vi "get_averaging_params_fd.vi"(10 "Modulation info":T3 {"Hi channels at low" min=0 step=1; "Low carriers" format="%#_6p"; "High carriers" format="%#_6p"}, 11 "Config":T4={"I/O"={"Format"={"Rate"=4, "Bits"=32, "Channels"=2}, "card #"=1, "# buffers"=96000}, "High rate STFT"={"Win param"=101.5, "Window type"=61, "Win order"=2, "DFT size"=64, "Channels"=[7], "Oversample"=64}, "Low rate STFT"={"Win param"=120.0, "Window type"=61, "Win order"=8, "DFT size"=64, "Channels"=[7], "Oversample"=64}, "Filtering"={"Hum"={"Frequency"=0.0, "Tc"=0.0, "Limit"=101.5, "FFT filter"=FALSE, "Detrend mode"=enum."Robust linear", "Enable"=FALSE}, "Kalman"={"Process noise"=101.5, "Measure noise"=101.5, "Unlock m noise"=101.5, "Mode"=enum."FFT"}, "Distortion"={"LF cut"=101.5, "Tc"=3.0, "Limit"=101.5, "FFT filter"=FALSE, "Detrend mode"=enum."Robust linear", "Enable"=FALSE}, "Lowpass"={"Frequency"=0.0, "Order"=0, "Enable"=FALSE}, "Impulse"={"Win order"=102, "Locked limit"=101.5, "Locked count"=102, "Threshold Tc"=101.5, "Thresh sigmas"=101.5, "Thresh min"=101.5, "After"=0, "Detrend"=FALSE, "Enable"=FALSE}}} {"Filtering"."Impulse"."Thresh min" format="%#_3p"; "Filtering"."Impulse"."Threshold Tc" format="%#_3p"; "Filtering"."Impulse"."Locked limit" format="%#_3p"; "Filtering"."Impulse"."Thresh sigmas" format="%#_3p"; "Filtering"."Lowpass"."Frequency" format="%#_4p"; "Filtering"."Distortion"."Limit" format="%#_3p"; "Filtering"."Distortion"."LF cut" format="%#_3p"; "Filtering"."Kalman"."Unlock m noise" format="%#_3p"; "Filtering"."Kalman"."Measure noise" format="%#_3p"; "Filtering"."Kalman"."Process noise" format="%#_3p"; "Filtering"."Hum"."Limit" format="%#_3p"; "Filtering"."Hum"."Frequency" format="%#_4p"; "Low rate STFT"."Oversample" min=1 step=1; "Low rate STFT"."Channels" min=0 step=1; "Low rate STFT"."DFT size" min=1 step=1; "Low rate STFT"."Window type" items=["Rectangle"=0, "Hanning"=1, "Hamming"=2, "Blackman-Harris"=3, "Exact Blackman"=4, "Blackman"=5, "Flat Top"=6, "4 Term B-Harris "=7, "7 Term B-Harris"=8, "Low Sidelobe"=9, "Blackman Nuttall"=11, "Triangle"=30, "Bartlett-Hanning"=31, "Bohman"=32, "Parzen"=33, "Welch"=34, "Kaiser"=60, "Dolph-Chebyshev"=61, "Gaussian"=62]; "High rate STFT"."Oversample" min=1 step=1; "High rate STFT"."Channels" min=0 step=1; "High rate STFT"."DFT size" min=1 step=1; "High rate STFT"."Window type" items=["Rectangle"=0, "Hanning"=1, "Hamming"=2, "Blackman-Harris"=3, "Exact Blackman"=4, "Blackman"=5, "Flat Top"=6, "4 Term B-Harris "=7, "7 Term B-Harris"=8, "Low Sidelobe"=9, "Blackman Nuttall"=11, "Triangle"=30, "Bartlett-Hanning"=31, "Bohman"=32, "Parzen"=33, "Welch"=34, "Kaiser"=60, "Dolph-Chebyshev"=61, "Gaussian"=62]}) -> (2 "Hum params":T1={"Order"=0, "Time constant"=0.0, "Detrend mode"=enum."Robust linear", "TD amplitude limit"=inf, "FFT filter"=TRUE, "Notch channels"=[], "LF cutoff"=0, "FD amplitude limit"=0.0}, 3 "Distortion params":T1={"Order"=0, "Time constant"=0.0, "Detrend mode"=enum."Robust linear", "TD amplitude limit"=inf, "FFT filter"=TRUE, "Notch channels"=[], "LF cutoff"=0, "FD amplitude limit"=0.0})   [LabVIEW 2014]
uses:
  averaging_filter_params.ctl
  detrend_mode.ctl
  ilemt_config.ctl
  io_config.ctl
  stft_params.ctl
  <vilib>/Analysis/4window.llb/windowTd.ctl
  filter_params.ctl
  modulation_info.ctl
  <vilib>/Analysis/NI_AALPro.lvlib
panel:
  # "Get averaging filter parameters for the distortion and hum filters,\noperating at Fd demodulated output rate."
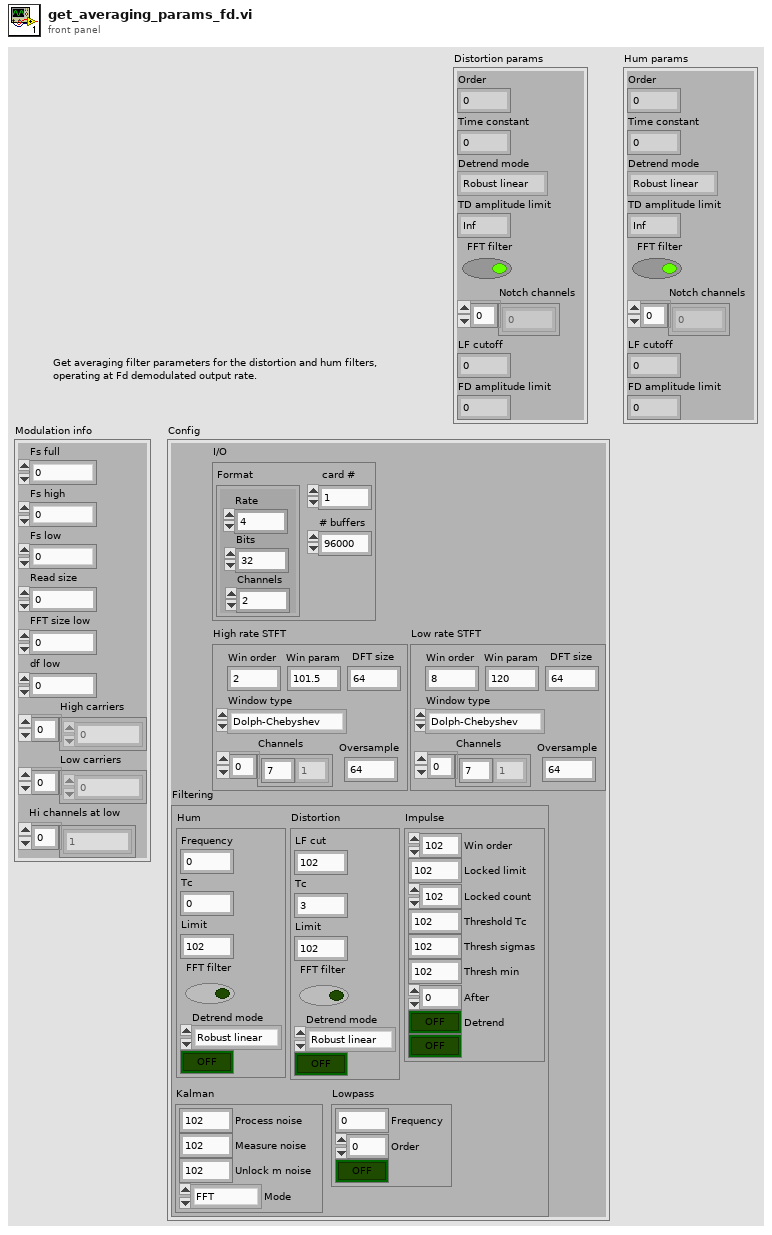
[diagram p1: front panel]
types:
  T1 = typedef "averaging_filter_params.ctl" = cluster{"Order":i32, "Time constant":dbl, "Detrend mode":T2, "TD amplitude limit":dbl, "FFT filter":bool, "Notch channels":i32[], "LF cutoff":i32, "FD amplitude limit":dbl}
  T2 = typedef "detrend_mode.ctl" = enum16{"Zero mean", "Linear", "Robust linear"}
  T3 = typedef "modulation_info.ctl" = cluster{"Fs full":dbl, "Fs high":dbl, "Fs low":dbl, "Read size":i32, "FFT size low":i32, "df low":dbl, "High carriers":dbl[], "Low carriers":dbl[], "Hi channels at low":i32[]}
  T4 = typedef "ilemt_config.ctl" = cluster{"I/O":T5, "High rate STFT":T6, "Low rate STFT":T6, "Filtering":T8}
  T5 = typedef "io_config.ctl" = cluster{"Format":cluster{"Rate":i32, "Bits":i32, "Channels":u32}, "card #":u32, "# buffers":i32}
  T6 = typedef "stft_params.ctl" = cluster{"Win param":dbl, "Window type":T7, "Win order":i32, "DFT size":i32, "Channels":i32[], "Oversample":i32}
  T7 = typedef "NI_AALPro.lvlib/windowTd.ctl" = u32
  T8 = typedef "filter_params.ctl" = cluster{"Hum":cluster{"Frequency":dbl, "Tc":dbl, "Limit":dbl, "FFT filter":bool, "Detrend mode":T2, "Enable":bool}, "Kalman":cluster{"Process noise":dbl, "Measure noise":dbl, "Unlock m noise":dbl, "Mode":enum16{"FFT", "KF demod"}}, "Distortion":cluster{"LF cut":dbl, "Tc":dbl, "Limit":dbl, "FFT filter":bool, "Detrend mode":T2, "Enable":bool}, "Lowpass":cluster{"Frequency":dbl, "Order":i32, "Enable":bool}, "Impulse":cluster{"Win order":i32, "Locked limit":dbl, "Locked count":i32, "Threshold Tc":dbl, "Thresh sigmas":dbl, "Thresh min":dbl, "After":i32, "Detrend":bool, "Enable":bool}}
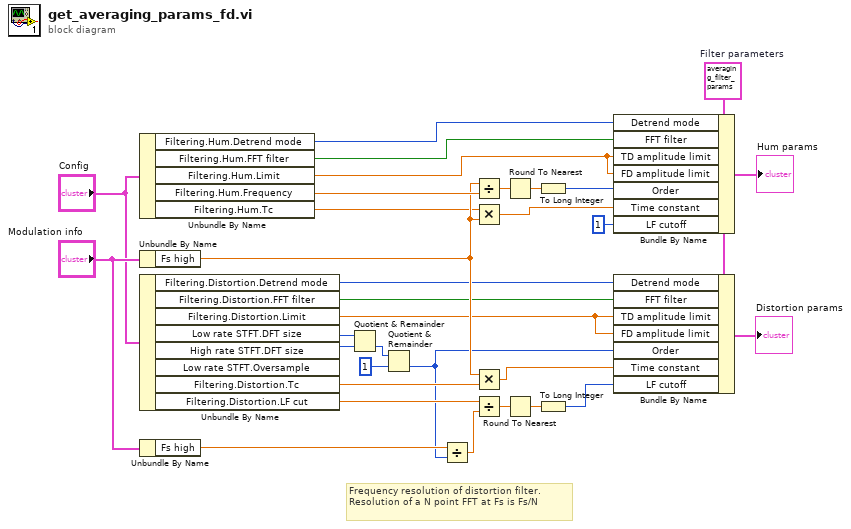
[diagram p0: block diagram]
diagram:
  w15 = T1 {"Order"=0, "Time constant"=0.0, "Detrend mode"=enum."Robust linear", "TD amplitude limit"=inf, "FFT filter"=TRUE, "Notch channels"=[], "LF cutoff"=0, "FD amplitude limit"=inf}  # Filter parameters
  # "Frequency resolution of distortion filter.   Resolution of a N point FFT at Fs is Fs/N"
  n1 = Unbundle By Name("Config") -> ("Filtering.Hum.Detrend mode"=w7:T2, "Filtering.Hum.FFT filter"=w8:bool, "Filtering.Hum.Limit"=w9:dbl, "Filtering.Hum.Frequency"=w30:dbl, "Filtering.Hum.Tc"=w18:dbl)
  n2 = Unbundle By Name("Modulation info") -> ("Fs high"=w26:dbl)
  n3 = Unbundle By Name("Config") -> ("Filtering.Distortion.Detrend mode"=w5:T2, "Filtering.Distortion.FFT filter"=w4:bool, "Filtering.Distortion.Limit"=w6:dbl, "Low rate STFT.DFT size"=w14:i32, "High rate STFT.DFT size"=w13:i32, "Filtering.Distortion.Tc"=w27:dbl, "Filtering.Distortion.LF cut"=w22:dbl)  [unwired: 1 out]
  n4 = Unbundle By Name("Modulation info") -> ("Fs high"=w11:dbl)
  n5 = Quotient & Remainder(x=w14, y=w13) -> (floor(x/y)=w3:i32)  [unwired: 1 out]
  n6 = Quotient & Remainder(x=w3, y=1) -> (floor(x/y)=w2:i32)  [unwired: 1 out]
  n7 = Divide(x=w11, y=w2) -> (x/y=w10:dbl)
  n8 = Divide(x=w26, y=w30) -> (x/y=w17:dbl)
  n9 = Multiply(x=w18, y=w26) -> (x*y=w25:dbl)
  n10 = Multiply(x=w26, y=w27) -> (x*y=w24:dbl)
  n11 = Divide(x=w22, y=w10) -> (x/y=w31:dbl)
  n12 = Round To Nearest(number=w17) -> (nearest integer value=w19:dbl)
  n13 = Round To Nearest(number=w31) -> (nearest integer value=w32:dbl)
  n14 = To Long Integer(number=w19) -> (32bit integer=w20:i32)
  n15 = To Long Integer(number=w32) -> (32bit integer=w28:i32)
  n16 = Bundle By Name(cluster=w15, "Detrend mode"=w7, "FFT filter"=w8, "TD amplitude limit"=w9, "FD amplitude limit"=w9, "Order"=w20, "Time constant"=w25, "LF cutoff"=1) -> (→"Hum params":T1)
  n17 = Bundle By Name(cluster=w15, "Detrend mode"=w5, "FFT filter"=w4, "TD amplitude limit"=w6, "FD amplitude limit"=w6, "Order"=w2, "Time constant"=w24, "LF cutoff"=w28) -> (→"Distortion params":T1)
